vi "medicaoIXV.vi"() -> ()   [LabVIEW 2012]
uses:
  <vilib>/Utility/file.llb/Write To Spreadsheet File (string).vi
  <vilib>/Utility/file.llb/Write To Spreadsheet File (DBL).vi
  <instrlib>/Agilent 6XXX Series/Agilent 6XXX Series.lvlib
panel:
  out "array":dbl[][](array[numeric])
  in  "Tab Control":enum32{"Entrada de dados", "Saída de dados"}(tab)
  out "ON/OFF":bool
  in  "Pontos":dbl
  in  "Tensão máxima":dbl
  in  "Nome da célula":string
  in  "Local":path
  in  "Delay(ms)":dbl
  in  "Start":bool
  in  "Print Screen":bool
  out "IXV":cluster{"Y":dbl[], "Y":dbl[]}[](graph)
  out "output voltage":dbl
  out "Tensao Atual":dbl
  out "Corrente Atual":dbl
  out "Ponto Atual":i32
  out "TABELA DE DADOS\nTensão(fonte)     Tensão                  Corrente            Pontos":dbl[][](array[numeric]) caption="all rows" format="%0.3f"
  in  "stop":bool
  in  "CorrenteGraph":dbl
  in  "error in (no error)":errorcluster
  out "error out":errorcluster
  in  "TensaoGraph":dbl
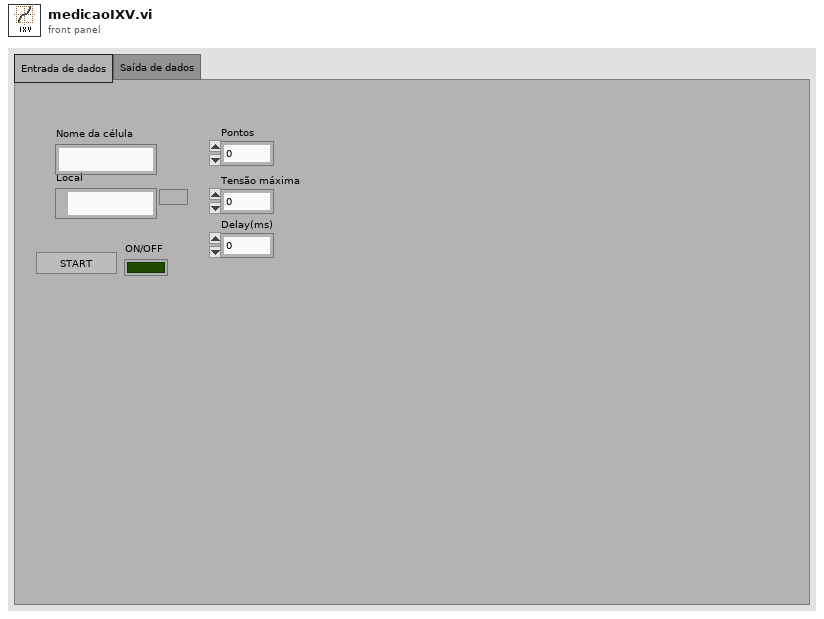
[diagram p1: front panel]
types:
  T1 = typedef "imagedata.ctl" = cluster{"image type":i32, "image depth":i32, "image":u8[], "mask":u8[], "colors":u32[], "Rectangle":cluster{"left":i16, "top":i16, "right":i16, "bottom":i16}}
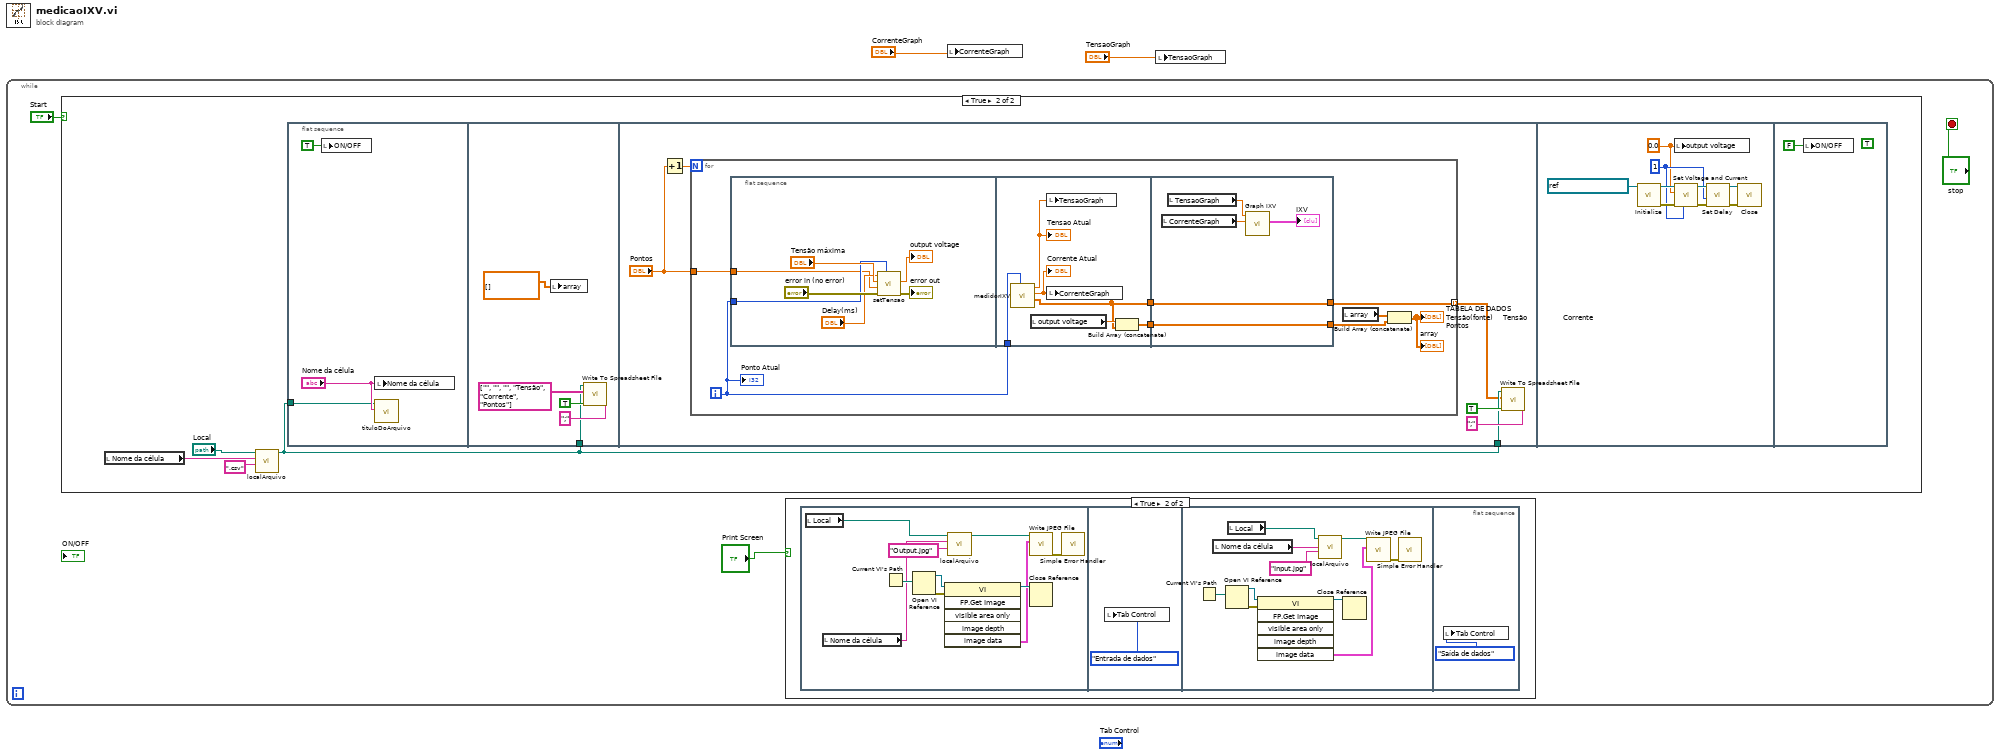
[diagram p0: block diagram]
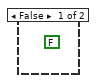
[diagram p3: hidden frame]
diagram:
  n1 = while {
    stop <- "stop" stop-if-true
    n2 = case shown="True" "Start" {
      frame False {
        (unwired) FALSE
      }
      frame True {
        n3 = local read "Nome da célula"() -> (w28:string)
        n4 = call "localArquivo.vi"("extensão"=".csv", "Nome do arquivo"=w28, "Local"="Local") -> ("Path"=w30:path)  [unwired: 8 in]
        n5 = flat-sequence {
          tunnel: w30 -> [w33]
          tunnel: w30 -> [w36]
          tunnel: w30 -> [w43]
          frame #0 {
            n6 = local write "ON/OFF"(TRUE ("ON/OFF")) -> ()
            n7 = local write "Nome da célula"("Nome da célula") -> ()
            n8 = call "tituloDoArquivo.vi"("Nome da célula"="Nome da célula", "file path (dialog if empty)"=w33) -> ()  [unwired: 10 in]
          }
          frame #1 {
            n9 = local write "array"(dbl[][] [] ("array")) -> ()
            n10 = call-poly <vilib>:"Write To Spreadsheet File.vi"("delimiter (\\t)"=";" ("delimiter (\\t)"), "append to file? (new file:F)"=TRUE, "2D data"=string[][] [["", "", ""], ["Tensão", "Corrente", "Pontos"]], "file path (dialog if empty)"=w36) -> ()  [unwired: 4 in, 1 out]
          }
          frame #2 {
            n11 = Increment(x="Pontos") -> (x+1=w42:dbl)
            n12 = for {
              N: w42 -> [_]
              tunnel: [w51] -> w40 mode=indexing
              tunnel: "Pontos" -> [w53]
              i -> [w52]
              n13 = flat-sequence {
                tunnel: w53 -> [w56]
                tunnel: w52 -> [w57]
                tunnel: w52 -> [w66]
                tunnel: [w61] -> w50
                tunnel: [w63] -> w49
                tunnel: [w70] -> w48
                tunnel: [w71] -> w51
                tunnel: w50 -> [w71]
                tunnel: w49 -> [w70]
                frame #0 {
                  n14 = call "setTensao.vi"("Ponto"=w57, "error in (no error)"="error in (no error)", "Pontos"=w56, "Tensão máxima"="Tensão máxima", "delay(ms)"="Delay(ms)") -> ("error out"=→"error out":errorcluster, "output voltage"=→"output voltage":dbl)  [unwired: 5 in]
                }
                frame #1 {
                  n15 = call "medidorIXV.vi"("Ponto"=w66) -> ("Array"=w61:dbl[], "Corrente Atual"=w65:dbl, "Tensao Atual"=w64:dbl)  [unwired: 8 in]
                  "Corrente Atual" <- w65
                  "Tensao Atual" <- w64
                  n16 = local read "output voltage"() -> (w62:dbl)
                  n17 = local write "TensaoGraph"(w64) -> ()
                  n18 = local write "CorrenteGraph"(w65) -> ()
                  n19 = Build Array (concatenate)(w62, w61) -> (w63:dbl[])
                }
                frame #2 {
                  n20 = local read "CorrenteGraph"() -> (w67:dbl)
                  n21 = local read "TensaoGraph"() -> (w68:dbl)
                  n22 = call "Graph IXV"("Y Input"=w67, "X Input"=w68) -> ("XY Graph"=→"IXV":cluster{"Y":dbl[], "Y":dbl[]}[])  [unwired: 3 in, 6 out]
                }
              }
              n23 = local read "array"() -> (w47:dbl[][])
              n24 = Build Array (concatenate)(w47, w48) -> (→"TABELA DE DADOS\nTensão(fonte)     Tensão                  Corrente            Pontos" →"array":dbl[][])
              "Ponto Atual" <- w52
            }
            n25 = call-poly <vilib>:"Write To Spreadsheet File.vi"("delimiter (\\t)"=";" ("delimiter (\\t)"), "append to file? (new file:F)"=TRUE, "2D data"=w40, "file path (dialog if empty)"=w43) -> ()  [unwired: 4 in, 1 out]
          }
          frame #3 {
            w72 = 0.0 ("voltage (0 V)")
            w75 = u8 1 ("channel (1)")
            n26 = call <instrlib>:"Initialize.vi"("VISA resource name"=refnum<visa-resource-name> "GPIB0::5::INSTR") -> ("error out"=w77:errorcluster, "VISA resource name out"=w76:refnum<visa-resource-name>)  [unwired: 9 in]
            n27 = local write "output voltage"(w72) -> ()
            n28 = call <instrlib>:"Set Voltage and Current.vi"("channel (1)"=w75, "error in (no error)"=w77, "voltage (0 V)"=w72, "VISA resource name"=w76) -> ("error out"=w78:errorcluster, "VISA resource name out"=w79:refnum<visa-resource-name>)  [unwired: 6 in]
            n29 = call <instrlib>:"Set Delay.vi"("error in (no error)"=w78, "channel (1)"=w75, "VISA resource name"=w79) -> ("error out"=w73:errorcluster, "VISA resource name out"=w74:refnum<visa-resource-name>)  [unwired: 7 in]
            n30 = call <instrlib>:"Close.vi"("error in (no error)"=w73, "VISA resource name"=w74) -> ()  [unwired: 9 in, 1 out]
          }
          frame #4 {
            (unwired) TRUE
            n31 = local write "ON/OFF"(FALSE) -> ()
          }
        }
      }
    }
    n32 = case shown="True" "Print Screen" {
      frame False {
      }
      frame True {
        n33 = flat-sequence {
          frame #0 {
            n34 = local read "Local"() -> (w7:path)
            n35 = local read "Nome da célula"() -> (w6:string)
            n36 = Current VI's Path() -> (path=w12:path)
            n37 = Open VI Reference(vi path=w12) -> (vi reference=w13:refnum<vi>, error out=w14:errorcluster)  [unwired: 5 in]
            n38 = invoke class="VI" method="FP.Get Image"(reference=w13, error in=w14) -> (reference out=w11:refnum<vi>, "image data"=w10:T1)  [unwired: 4 in, 4 out]
            n39 = call "localArquivo.vi"("extensão"="Output.jpg", "Nome do arquivo"=w6, "Local"=w7) -> ("Path"=w15:path)  [unwired: 8 in]
            n40 = call <vilib>:"Write JPEG File.vi"("image data"=w10, "path to JPEG file"=w15) -> ("error out"=w9:errorcluster)  [unwired: 8 in, 1 out]
            n41 = Close Reference(reference=w11) -> ()  [unwired: 1 in, 1 out]
            n42 = call <vilib>:"Simple Error Handler.vi"("error in (no error)"=w9) -> ()  [unwired: 4 in, 5 out]
          }
          frame #1 {
            n43 = local write "Tab Control"(enum32{"Entrada de dados", "Saída de dados"}."Entrada de dados" ("Tab Control")) -> ()
          }
          frame #2 {
            n44 = Current VI's Path() -> (path=w25:path)
            n45 = local read "Nome da célula"() -> (w18:string)
            n46 = Open VI Reference(vi path=w25) -> (vi reference=w24:refnum<vi>, error out=w23:errorcluster)  [unwired: 5 in]
            n47 = local read "Local"() -> (w17:path)
            n48 = invoke class="VI" method="FP.Get Image"(reference=w24, error in=w23) -> (reference out=w26:refnum<vi>, "image data"=w21:T1)  [unwired: 4 in, 4 out]
            n49 = call "localArquivo.vi"("extensão"="Input.jpg", "Nome do arquivo"=w18, "Local"=w17) -> ("Path"=w20:path)  [unwired: 8 in]
            n50 = Close Reference(reference=w26) -> ()  [unwired: 1 in, 1 out]
            n51 = call <vilib>:"Write JPEG File.vi"("image data"=w21, "path to JPEG file"=w20) -> ("error out"=w22:errorcluster)  [unwired: 8 in, 1 out]
            n52 = call <vilib>:"Simple Error Handler.vi"("error in (no error)"=w22) -> ()  [unwired: 4 in, 5 out]
          }
          frame #3 {
            n53 = local write "Tab Control"(enum32{"Entrada de dados", "Saída de dados"}."Saída de dados" ("Tab Control")) -> ()
          }
        }
      }
    }
  }
  n54 = local write "CorrenteGraph"("CorrenteGraph") -> ()
  n55 = local write "TensaoGraph"("TensaoGraph") -> ()
